vi "MM_Module_Control.vi"(5 "MM_Module_Ctrlr_Mode":T2, 7 "Module Name":string, 8 "error in":errorcluster, 9 "Reset Module Names on Init":bool, 10 "Module_Names_Initial":string[](array[string]), 11 "MM_Module_Action In":T1) -> (0 "error out":errorcluster, 1 "Module_Actions_Current":T1[](array[typedef]), 2 "Module_Names_Current":string[](array[string]), 3 "MM_Module_Action Out":T1)   [LabVIEW 2018]
doc: "Used as a smart VIGlobal to manage startup, run, idle and exit of Module control loops. The VIG uses methods (Actions) to:\n 1. Initialize a list of Module names\n 2. Idle a named Module Loop\n 3. Start a Module, this is one time, returns to Idle after Module finishes\n 4. Run, this is a continous, repeated operation, until Idle or Exit is set.\n\nThe Controler Mode control is the normal Get-Set options. Each subloop in the system should have it's loop name added before Sets & Gets are performed. This allows multiple Modules to be added to the system and each Module to set it's own private subloops.\n\n2007_11 Mike Ashe\nmichael.ashe@imaginatics.net\nCell: 860-961-0876"
uses:
  MM_Module_Action.ctl
  MM_Module_Control_Mode.ctl
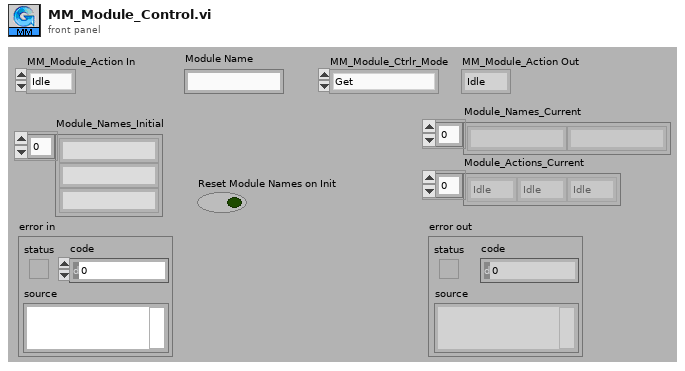
[diagram p1: front panel]
types:
  T1 = typedef "MM_Module_Action.ctl" = enum16{"Idle", "Start", "Run", "Exit"}
  T2 = typedef "MM_Module_Control_Mode.ctl" = enum16{"Get", "Set", "Init", "Get Initial Modules", "Add"}
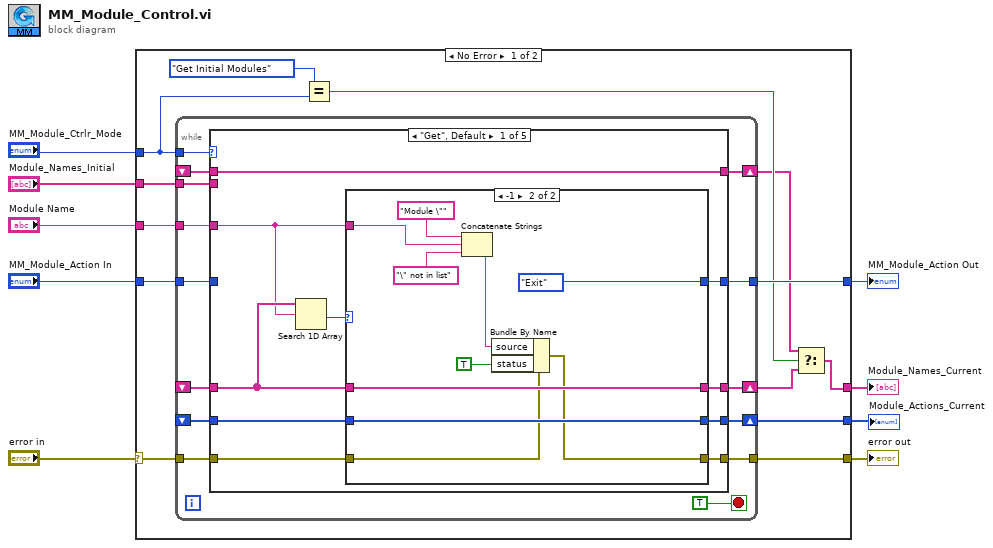
[diagram p0: block diagram]
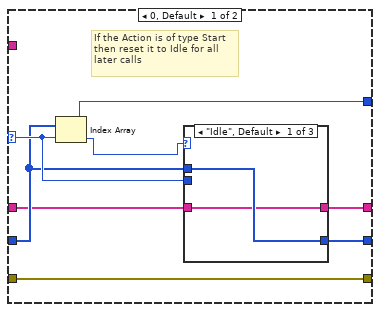
[diagram p2: hidden frame]
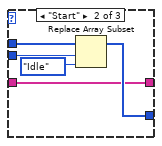
[diagram p3: hidden frame]
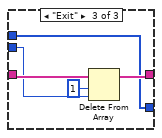
[diagram p4: hidden frame]
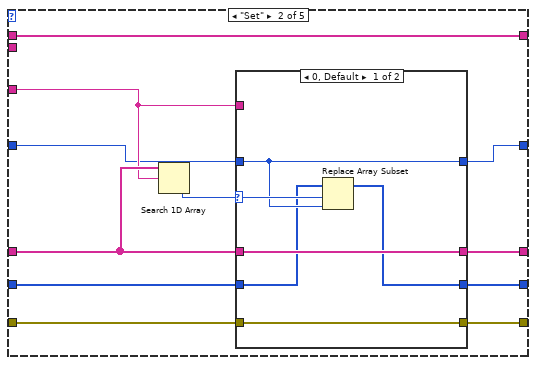
[diagram p5: hidden frame]
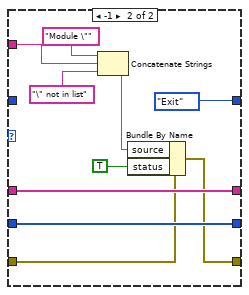
[diagram p6: hidden frame]
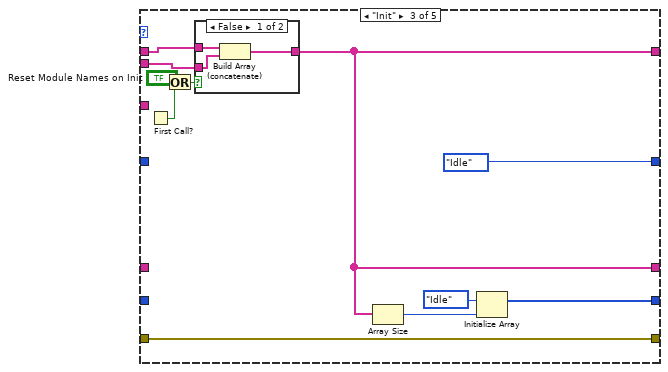
[diagram p7: hidden frame]
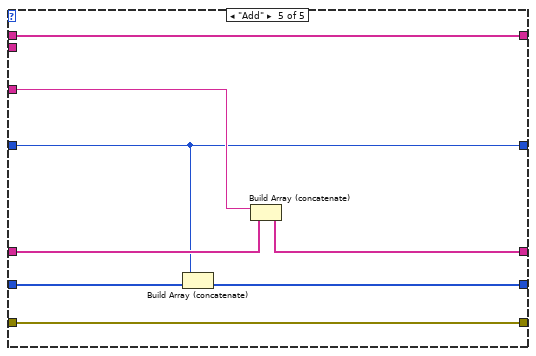
[diagram p10: hidden frame]
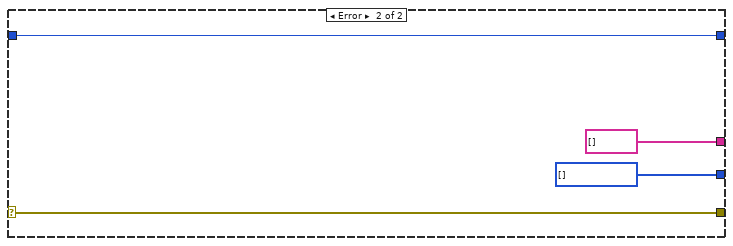
[diagram p11: hidden frame]
diagram:
  n1 = case shown="No Error" "error in" {
    selector: "error in" -> [w20 w134]
    tunnel: [w19 w134] -> w8
    tunnel: "MM_Module_Ctrlr_Mode" -> [w13 _]
    tunnel: "Module Name" -> [w22 _]
    tunnel: "Module_Names_Initial" -> [w14 _]
    tunnel: "MM_Module_Action In" -> [w21 w133]
    tunnel: [w18 w133] -> w4
    tunnel: [w15 string[] [] ("Module_Names_Initial")] -> w2
    tunnel: [w17 w131] -> w1
    frame No Error {
      n2 = while {
        shift-right: [w32] -> w16
        shift-left: _ -> [w35]
        tunnel: w13 -> [w36]
        tunnel: w22 -> [w34]
        tunnel: w21 -> [w31]
        tunnel: w20 -> [w29]
        tunnel: [w28] -> w19
        tunnel: [w27] -> w18
        shift-right: [w26] -> w17
        shift-left: _ -> [w25]
        shift-right: [w24] -> w10
        shift-left: _ -> [w33]
        tunnel: w14 -> [w23]
        stop <- TRUE stop-if-true
        n3 = case shown="\"Get\", Default" w36 {
          tunnel: w35 -> [w43 w83 _ w120 w130]
          tunnel: w34 -> [w40 w80 _ _ w127]
          tunnel: w33 -> [w37 w76 w106 w122 w123]
          tunnel: [w42 w82 w107 w120 w129] -> w32
          tunnel: w31 -> [_ w78 _ w121 w125]
          tunnel: w29 -> [w45 w85 w113 w118 w128]
          tunnel: [w38 w77 w113 w118 w128] -> w28
          tunnel: [w39 w79 MM_Module_Action."Idle" ("MM_Module_Action Out") w121 w125] -> w27
          tunnel: w25 -> [w44 w84 _ w119 w126]
          tunnel: [w41 w81 w109 w119 w124] -> w26
          tunnel: [w37 w76 w107 w122 w123] -> w24
          tunnel: w23 -> [_ _ w108 _ _]
          frame "Get", Default {
            n4 = Search 1D Array(1D array=w43, element=w40) -> (index of element=w46:i32)  [unwired: 1 in]
            n5 = case shown="-1" w46 {
              selector: w46 -> [w52 _]
              tunnel: w45 -> [w53 w73]
              tunnel: w44 -> [w51 w74]
              tunnel: w43 -> [w48 w75]
              tunnel: [w47 w75] -> w42
              tunnel: [w50 w74] -> w41
              tunnel: w40 -> [_ w69]
              tunnel: [w49 MM_Module_Action."Exit" ("MM_Module_Action Out")] -> w39
              tunnel: [w53 w67] -> w38
              frame 0, Default {
                # "If the Action is of type Start\nthen reset it to Idle for all\nlater calls"
                n6 = Index Array(array=w51, index=w52) -> (element=w49:T1)
                n7 = case shown="\"Idle\", Default" w49 {
                  tunnel: w52 -> [_ w60 w63]
                  tunnel: w51 -> [w55 w58 w61]
                  tunnel: [w55 w57 w61] -> w50
                  tunnel: [w54 w56 w65] -> w47
                  tunnel: w48 -> [w54 w56 w64]
                  frame "Idle", Default {
                  }
                  frame "Start" {
                    n8 = Replace Array Subset(array=w58, new element=MM_Module_Action."Idle" ("new element/subarray"), index=w60) -> (w57:T1[])
                  }
                  frame "Exit" {
                    n9 = Delete From Array(array=w64, length=1, index=w63) -> (array with subset deleted=w65:string[])  [unwired: 1 out]
                  }
                }
              }
              frame -1 {
                n10 = Concatenate Strings("Module \"" ("string"), w69, "\" not in list" ("string")) -> (w68:string)
                n11 = Bundle By Name(cluster=w73, "source"=w68, "status"=TRUE) -> (w67:errorcluster)
              }
            }
          }
          frame "Set" {
            n12 = Search 1D Array(1D array=w83, element=w80) -> (index of element=w86:i32)  [unwired: 1 in]
            n13 = case shown="0, Default" w86 {
              selector: w86 -> [w90 _]
              tunnel: w85 -> [w92 w100]
              tunnel: w84 -> [w88 w101]
              tunnel: w83 -> [w91 w102]
              tunnel: [w91 w102] -> w82
              tunnel: [w87 w101] -> w81
              tunnel: w80 -> [_ w96]
              tunnel: [w89 MM_Module_Action."Exit" ("MM_Module_Action Out")] -> w79
              tunnel: [w92 w94] -> w77
              tunnel: w78 -> [w89 _]
              frame 0, Default {
                n14 = Replace Array Subset(array=w88, new element=w89, index=w90) -> (w87:T1[])
              }
              frame -1 {
                n15 = Concatenate Strings("Module \"" ("string"), w96, "\" not in list" ("string")) -> (w95:string)
                n16 = Bundle By Name(cluster=w100, "source"=w95, "status"=TRUE) -> (w94:errorcluster)
              }
            }
          }
          frame "Init" {
            n17 = First Call?() -> (First Call?: T/F=w103:bool)
            n18 = Or(x="Reset Module Names on Init", y=w103) -> (x .or. y?=w104:bool)
            n19 = case shown="False" w104 {
              tunnel: w108 -> [w116 w117]
              tunnel: [w115 w117] -> w107
              tunnel: w106 -> [w114 _]
              frame False {
                n20 = Build Array (concatenate)(w114, w116) -> (w115:string[])
              }
              frame True {
              }
            }
            n21 = Array Size(array=w107) -> (size(s)=w110:i32)
            n22 = Initialize Array(MM_Module_Action."Idle" ("MM_Module_Action Out"), w110) -> (w109:T1[])
          }
          frame "Get Initial Modules" {
          }
          frame "Add" {
            n23 = Build Array (concatenate)(w125, w126) -> (w124:T1[])
            n24 = Build Array (concatenate)(w127, w130) -> (w129:string[])
          }
        }
      }
      n25 = Equal?(x=MM_Module_Control_Mode."Get Initial Modules" ("MM_Module_Ctrlr_Mode"), y=w13) -> (x = y?=w11:bool)
      n26 = Select(t=w10, s=w11, f=w16) -> (s? t:f=w15:string[])
    }
    frame Error {
      w131 = T1[] [] items=["Idle", "Start", "Run", "Exit"]
    }
  }
  "error out" <- w8
  "MM_Module_Action Out" <- w4
  "Module_Actions_Current" <- w1
  "Module_Names_Current" <- w2
